vi "微波探针下压同步采集系统.vi"() -> ()   [LabVIEW 2024]
uses:
  <vilib>/Analysis/Matrix/Datatypes/RealMatrix.ctl
  <vilib>/Instr/_visa.llb/VISA Configure Serial Port (Instr).vi
  <vilib>/Utility/file.llb/Write Delimited Spreadsheet (DBL).vi
  BP_GAS/GAS.lvlib
  BP_GAS/VIs/GA Open.vi
  BP_GAS/VIs/GA Reset.vi
  BP_GAS/VIs/GA Axis On.vi
  BP_GAS/VIs/GA Prf Trap.vi
  BP_GAS/VIs/GA Set Trap Prm Single.vi
  BP_GAS/VIs/GA Set Vel.vi
  BP_GAS/VIs/GA Set Pos.vi
  BP_GAS/VIs/GA Get Prf Pos.vi
  BP_GAS/VIs/GA Stop.vi
  BP_GAS/VIs/GA Update.vi
  <vilib>/Analysis/Matrix/NI_Matrix.lvlib
panel:
  out "循环次数":T1
  in  "循环次数":dbl
  out "步骤":T1
  in  "启用":bool
  in  "Real Matrix":T2 caption="顺序移动"
  out "U":dbl
  out "Z":dbl
  out "Y":dbl
  out "X":dbl
  out "错误输出 2":errorcluster caption="错误输出"
  out "错误输出":errorcluster
  out "电容":dbl(graph)
  out "电容表":dbl(knob) scale=0.0..20.0
  out "电容(F)":dbl
  out "损耗因子表":dbl(knob) scale=0.0..10.0
  out "损耗因子":dbl(graph)
  out "损耗因子(F)":dbl
  in  "测试参数":u16(ring) items=["Ls-Rs", "Cp-D"]
  in  "复位":bool
  out "运动状态":bool
  out "error out 2":errorcluster caption="error out"
  in  "停止运动":bool
  in  "开始运动":bool
  out "毫秒计时":u32
  out "时间":u32(graph)
  out "采集状态":bool
  out "位移 2":T3 scale=-10000.0..10000.0
  out "位置":dbl(graph)
  out "位置(pluse)":dbl
  out "info":string="打开成功！\r\n复位成功！\r\n轴使能成功！\r\n模式设置成功！\r\n参数设置成功！\r\n速度设置成功！\r\n目标位置成功！\r\n启动成功！\r\n启动成功！\r\n启动成功！\r\n启动成功！\r\n启动成功！\r\n启动成功！\r\n启动成功！\r\n启动成功！\r\n"
  out "实际位置":dbl
  in  "目标位置(mm or °)":dbl
  in  "设定速度(μm/s)":dbl=1.0 format="%#_13g"
  in  "轴号":i16=3
  out "电感":dbl(graph)
  out "电阻表 3":dbl(knob) scale=0.0..20.0
  out "电感(H)":dbl
  out "电阻表 2":dbl(knob) scale=0.0..10.0
  out "电阻":dbl(graph)
  out "电阻(Ω)":dbl
  in  "Baud Rate":u32=9600
  in  "LCR数字电桥":refnum<visa-resource-name>="COM7"
  in  "保存数据":bool
  in  "压力归零":bool
  in  "清除图表":bool
  in  "开始采集":bool
  out "压力表":dbl(knob) scale=0.0..20.0
  out "压力":dbl(graph)
  out "压力(g)":dbl
  in  "stop bits (10: 1 bit) 2":u16(ring)=10 caption="停止位（10: 1位）" items=["1.0"=10, "1.5"=15, "2.0"=20]
  in  "timeout (10sec) 2":u32=10000 caption="超时（10秒）"
  in  "parity (0:none) 2":enum16{"None", "Odd", "Even", "Mark", "Space"}(ring) caption="奇偶（0:无）"
  in  "baud rate (9600) 2":u32=9600 caption="波特率(9600)"
  in  "data bits (8) 2":u16=8 caption="数据比特(8)" min=5 max=8 step=1
  in  "VISA resource name 2":refnum<visa-resource-name>="COM5" caption="压力串口"
  in  "读取间隔（毫秒）":u32=100
  in  "停止":bool
  # "XYZU：0.078125μm/pluse"
  # "位置       速度     延时(ms)"
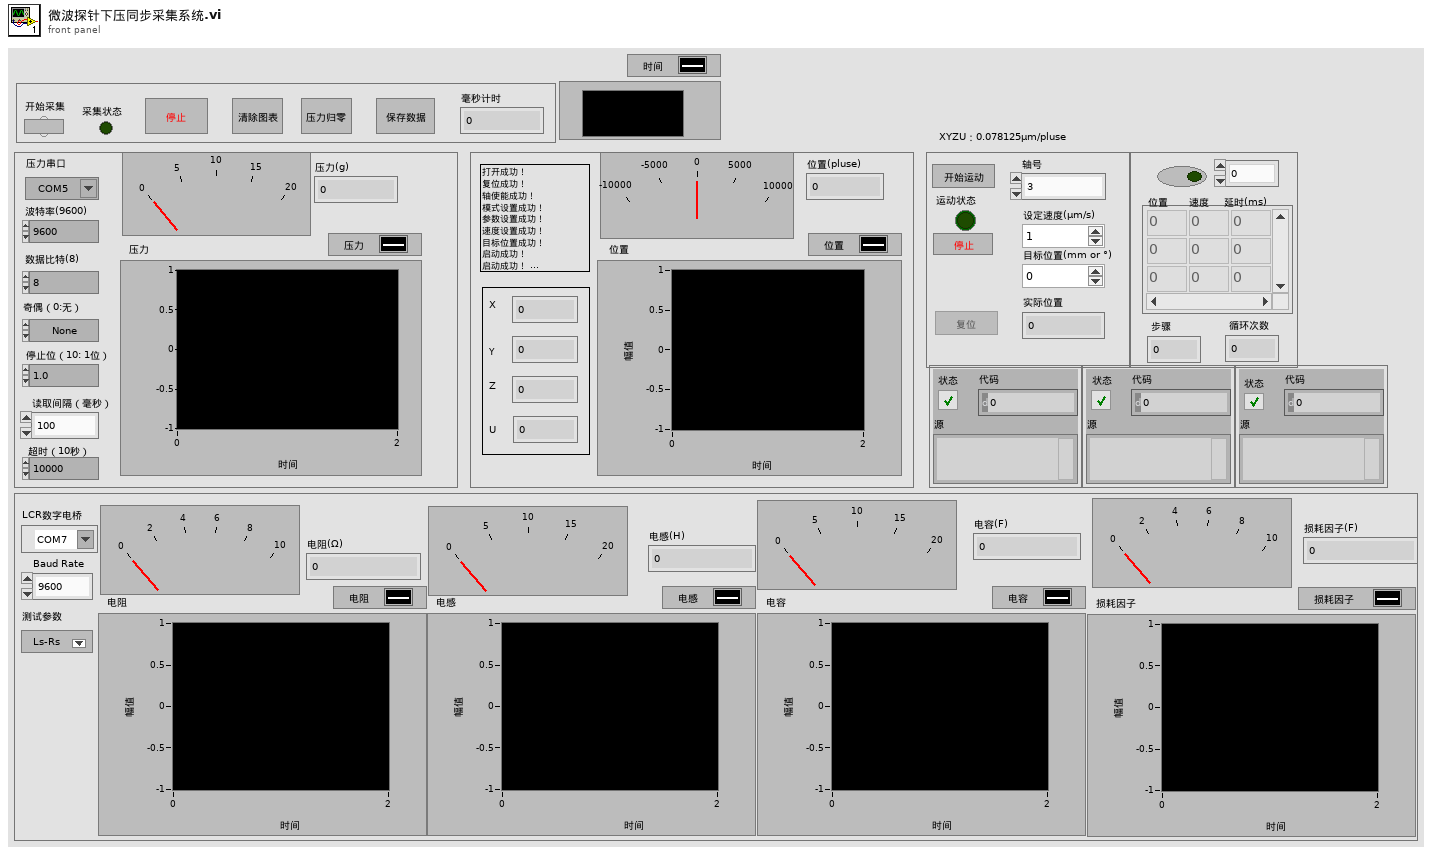
[diagram p1: front panel]
types:
  T1 = typedef "控件 3.ctl" = dbl
  T2 = typedef "NI_Matrix.lvlib/RealMatrix.ctl" = dbl[][]
  T3 = typedef "控件 1.ctl" = dbl
  T4 = enum8{"Enabled", "Disabled", "Disabled and Grayed Out"}
  T5 = cluster{"acc":dbl, "dec":dbl, "velStart":dbl, "smoothTime":i16}
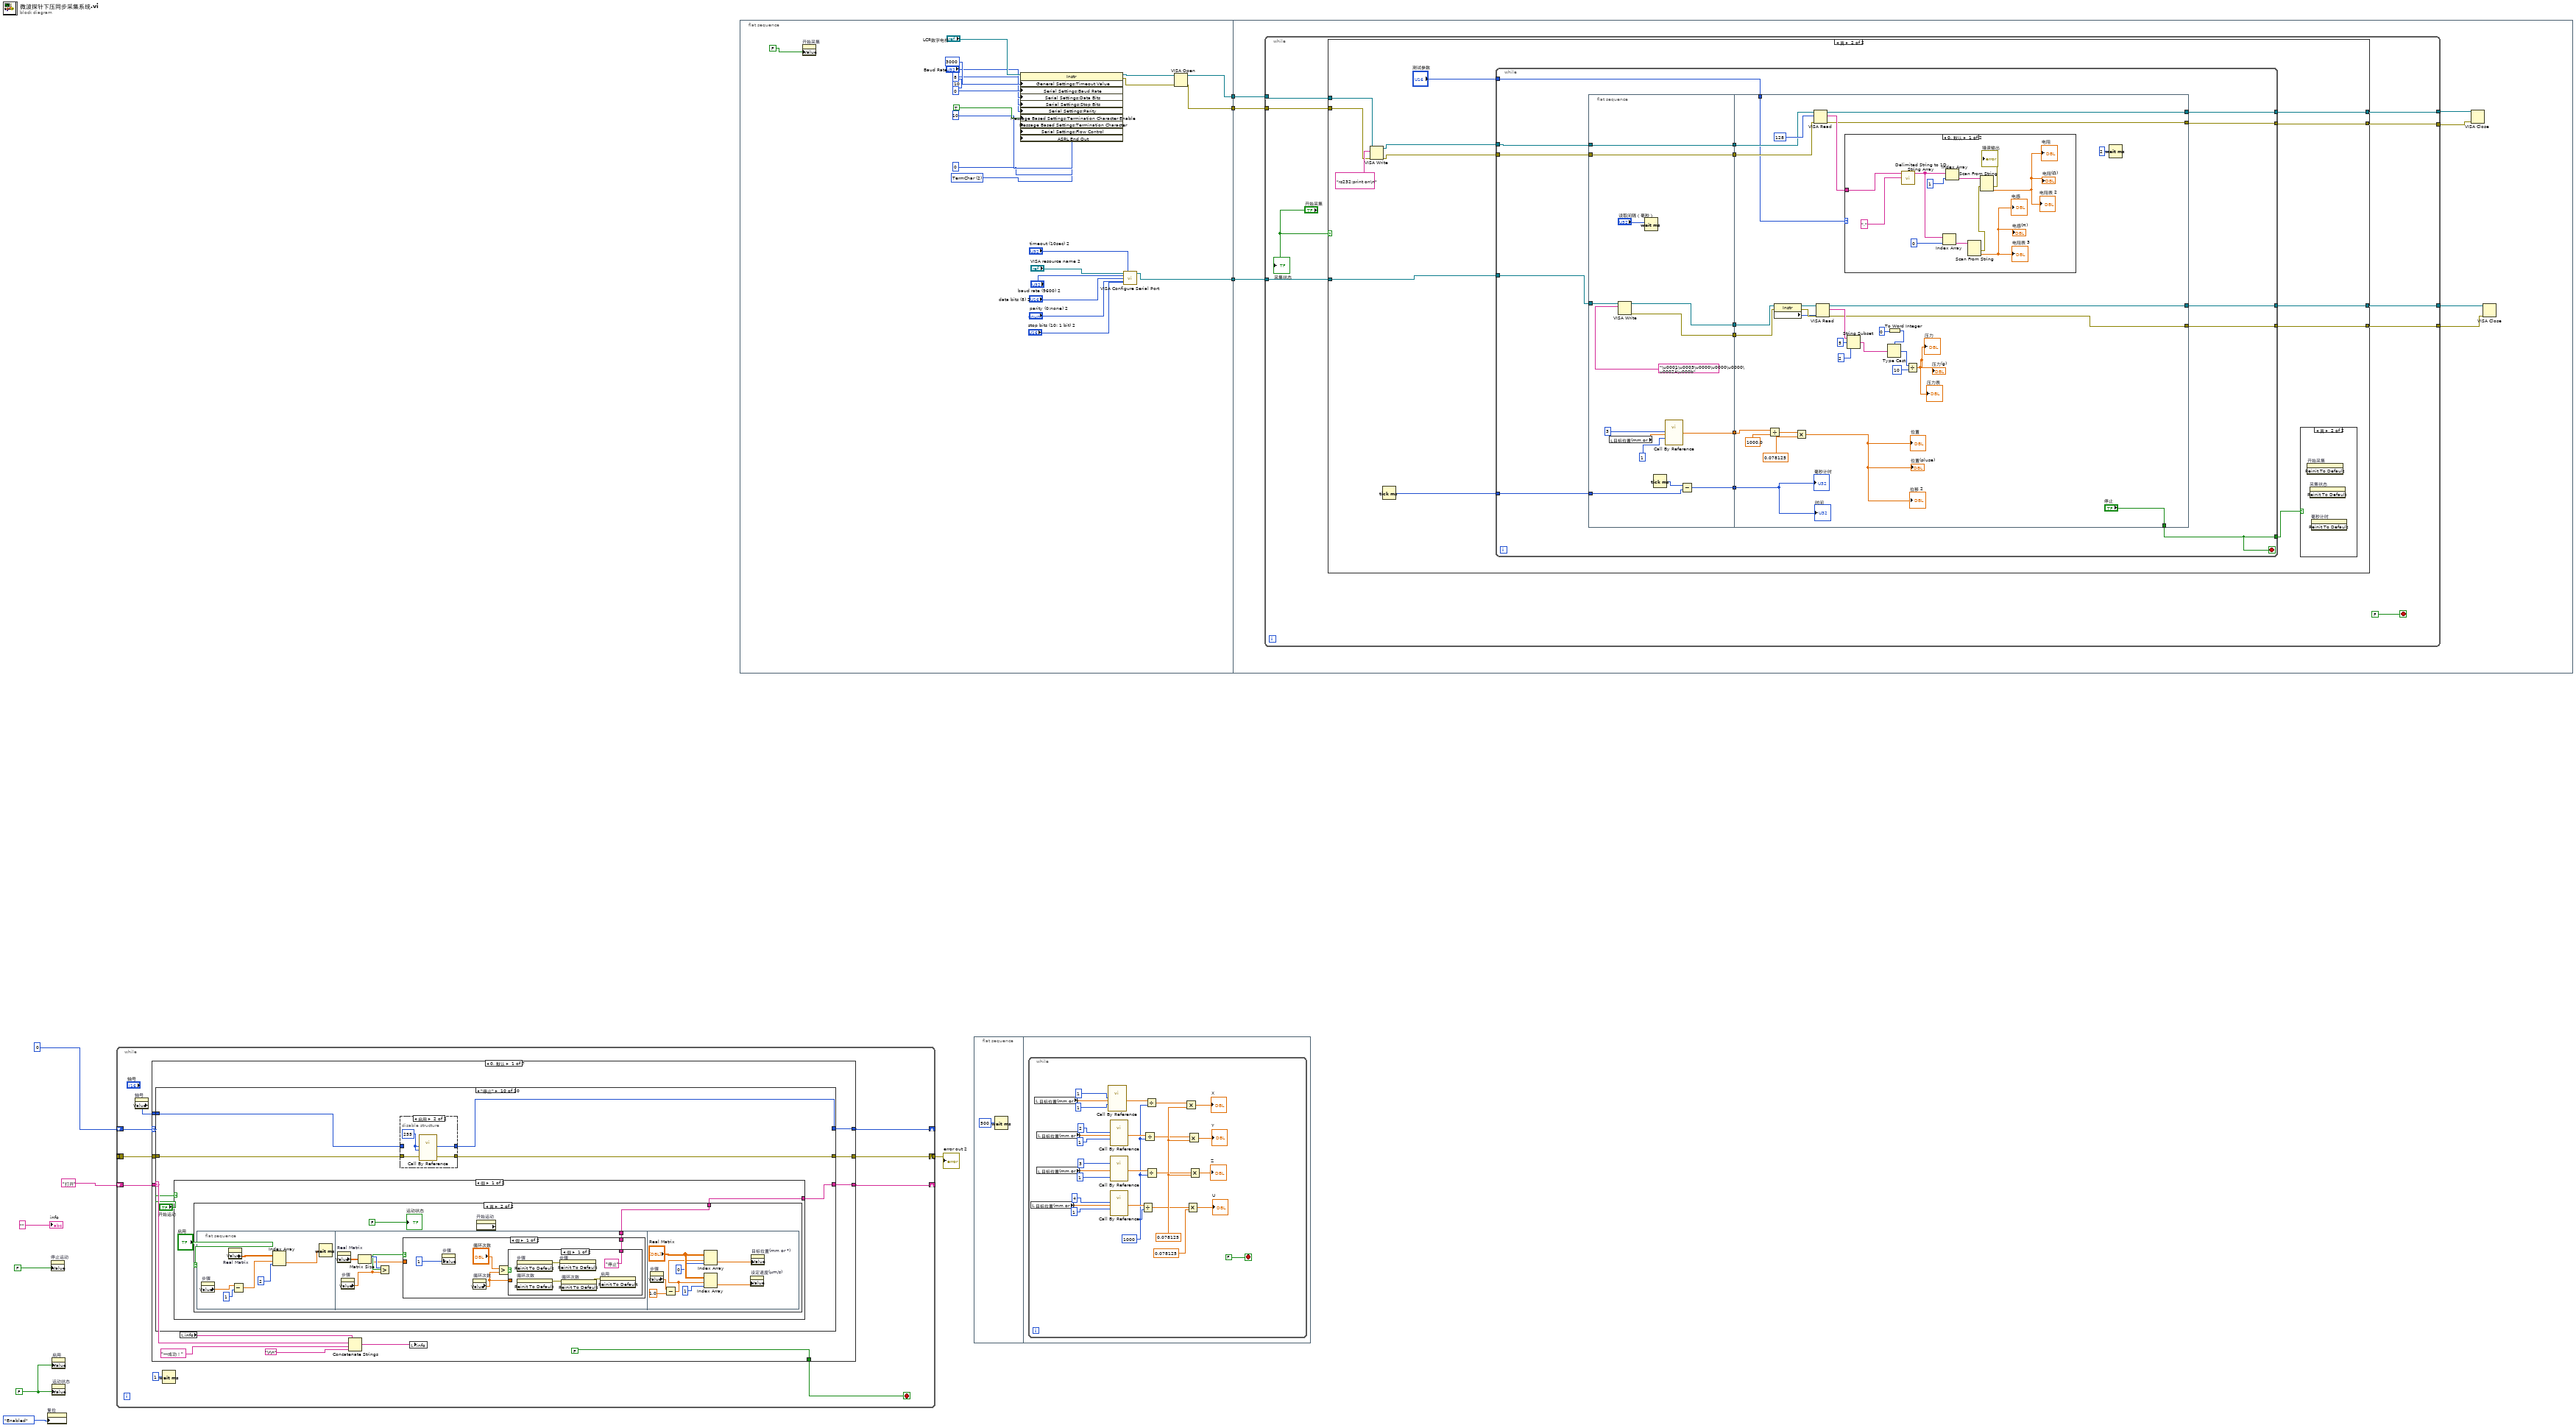
[diagram p0: block diagram]
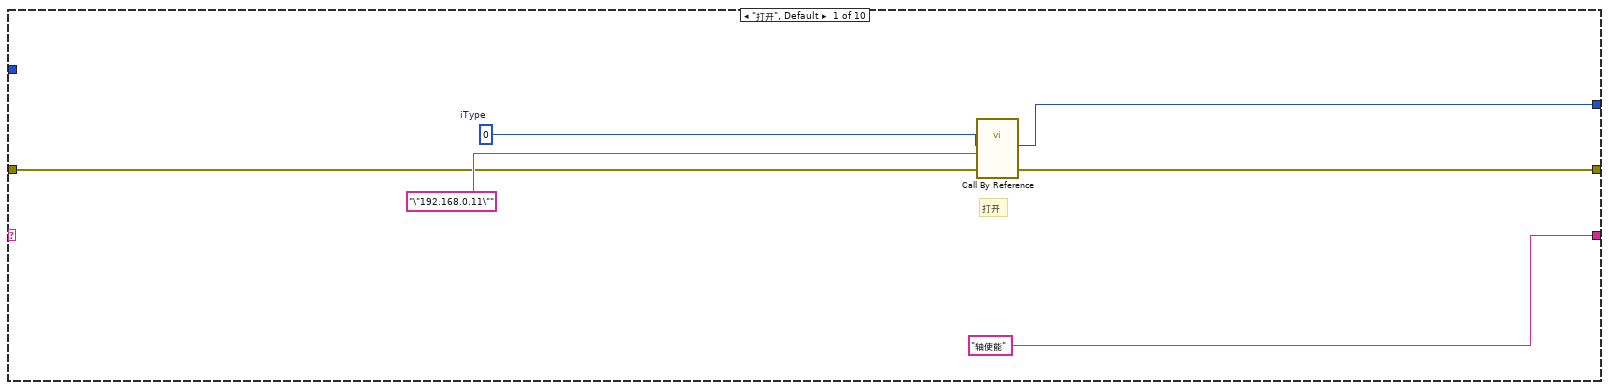
[diagram p2: hidden frame]
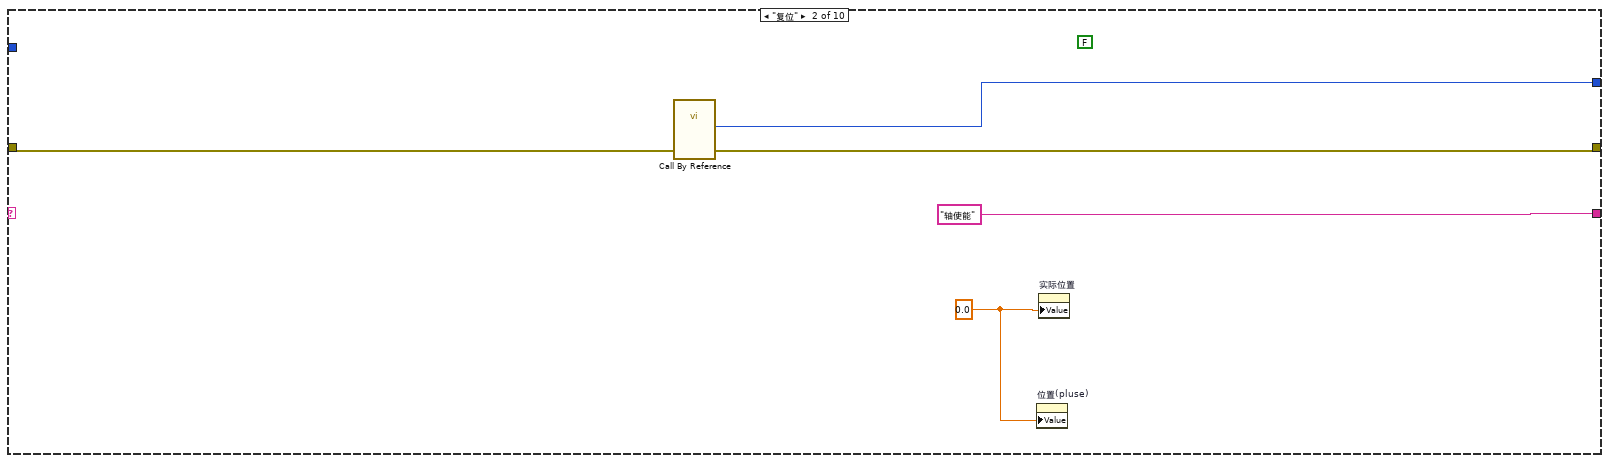
[diagram p3: hidden frame]
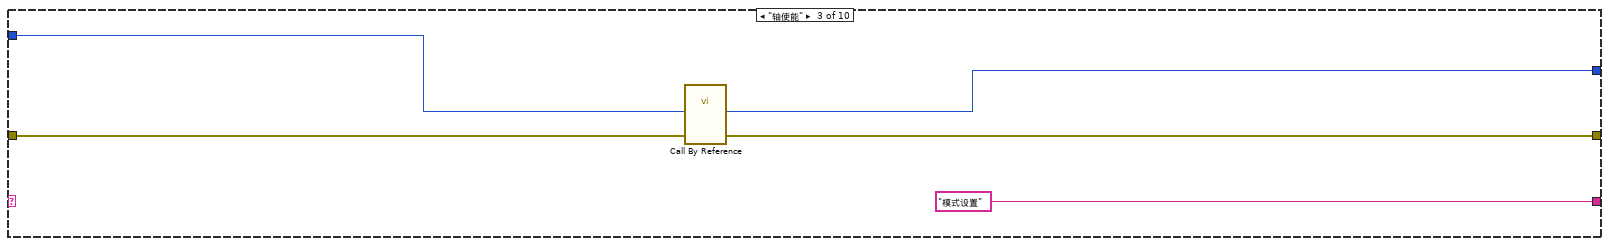
[diagram p4: hidden frame]
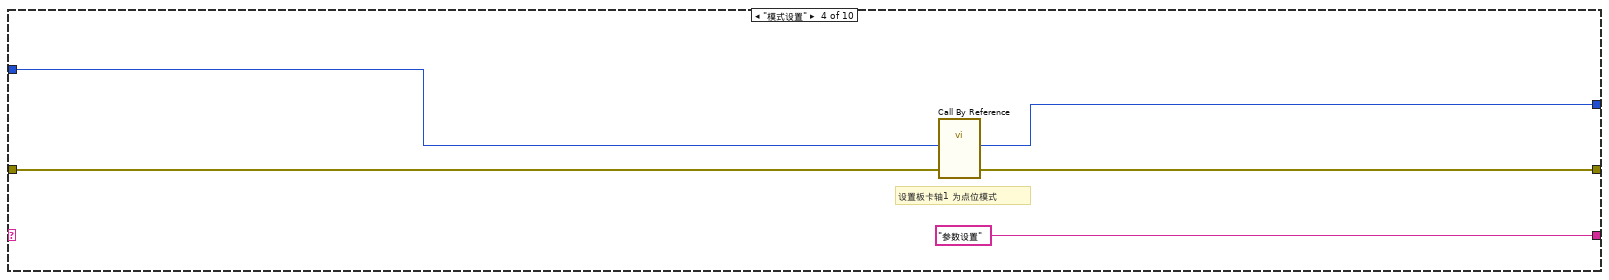
[diagram p5: hidden frame]
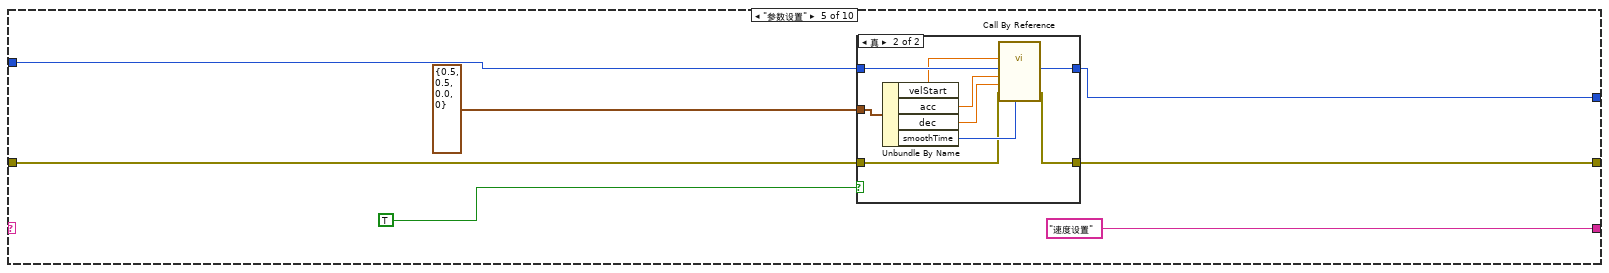
[diagram p6: hidden frame]
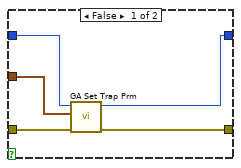
[diagram p7: hidden frame]
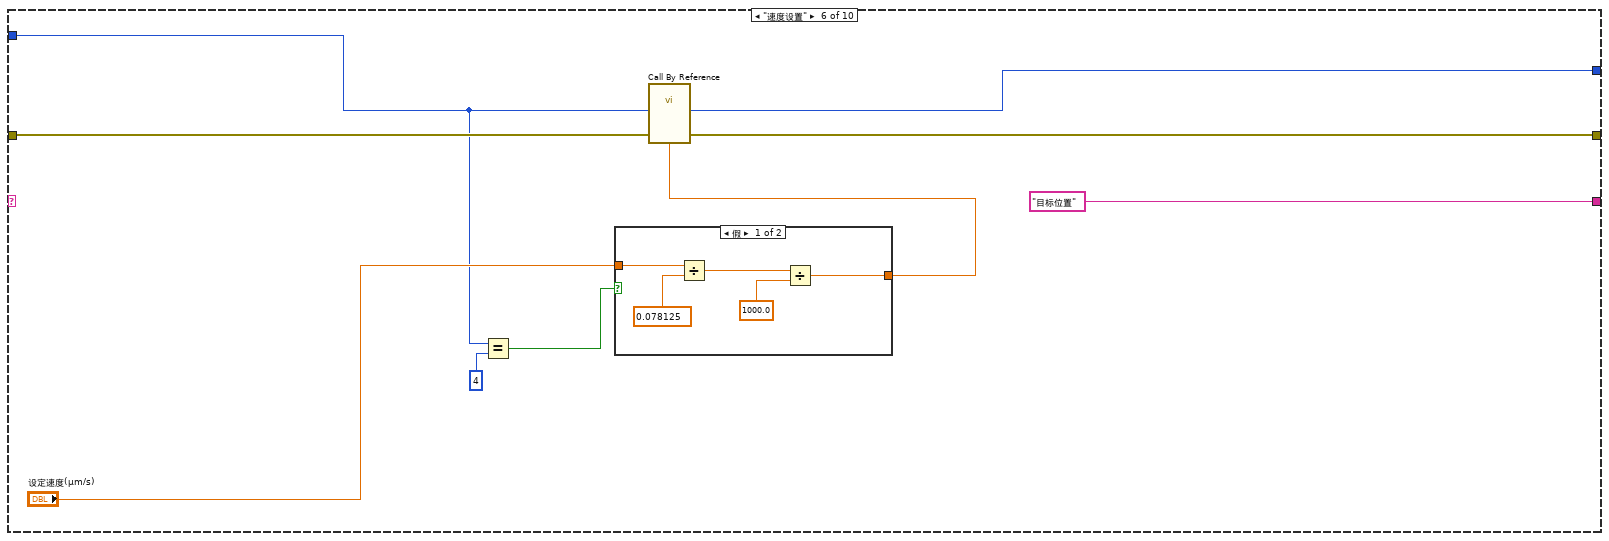
[diagram p8: hidden frame]
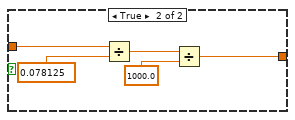
[diagram p9: hidden frame]
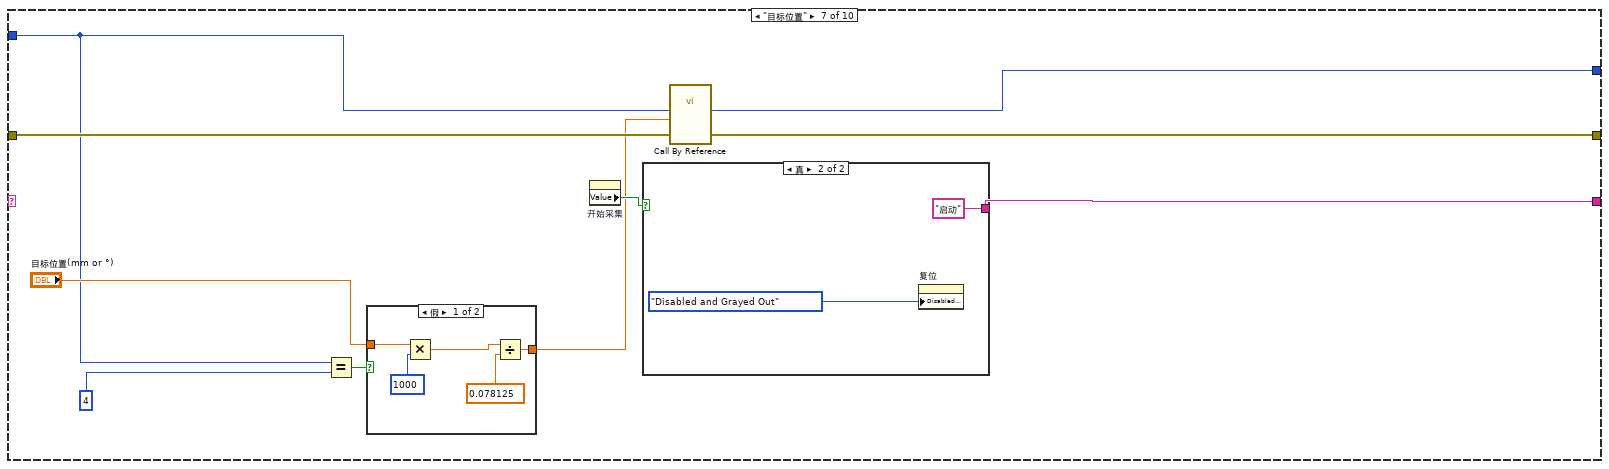
[diagram p10: hidden frame]
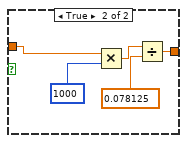
[diagram p11: hidden frame]
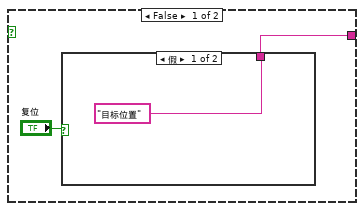
[diagram p12: hidden frame]
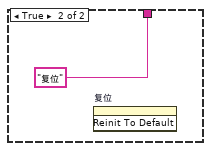
[diagram p13: hidden frame]
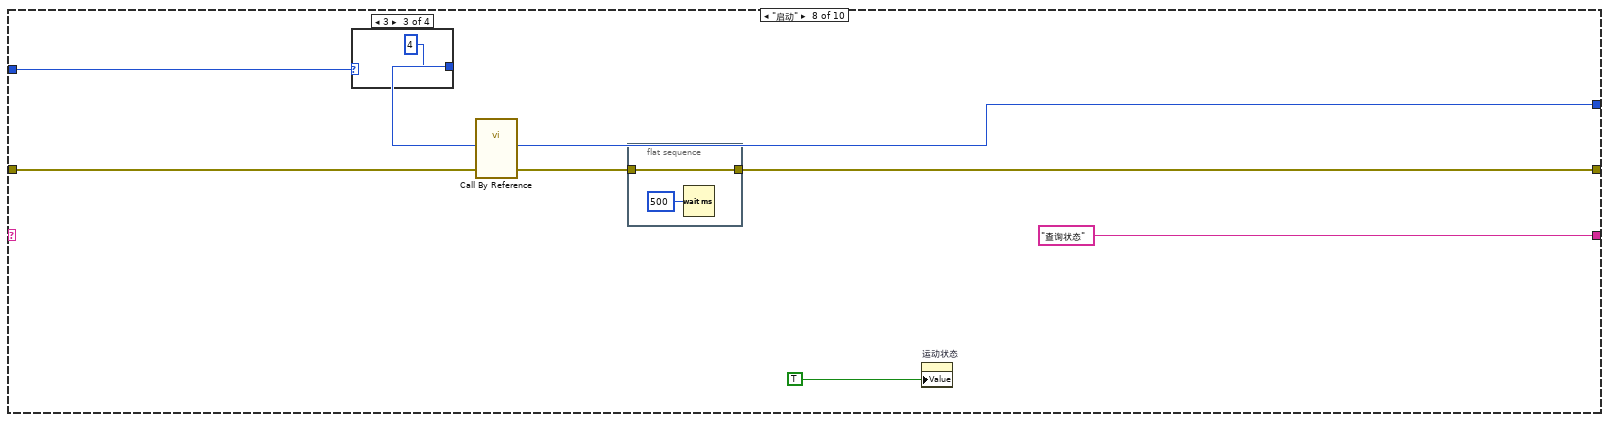
[diagram p14: hidden frame]
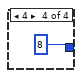
[diagram p17: hidden frame]
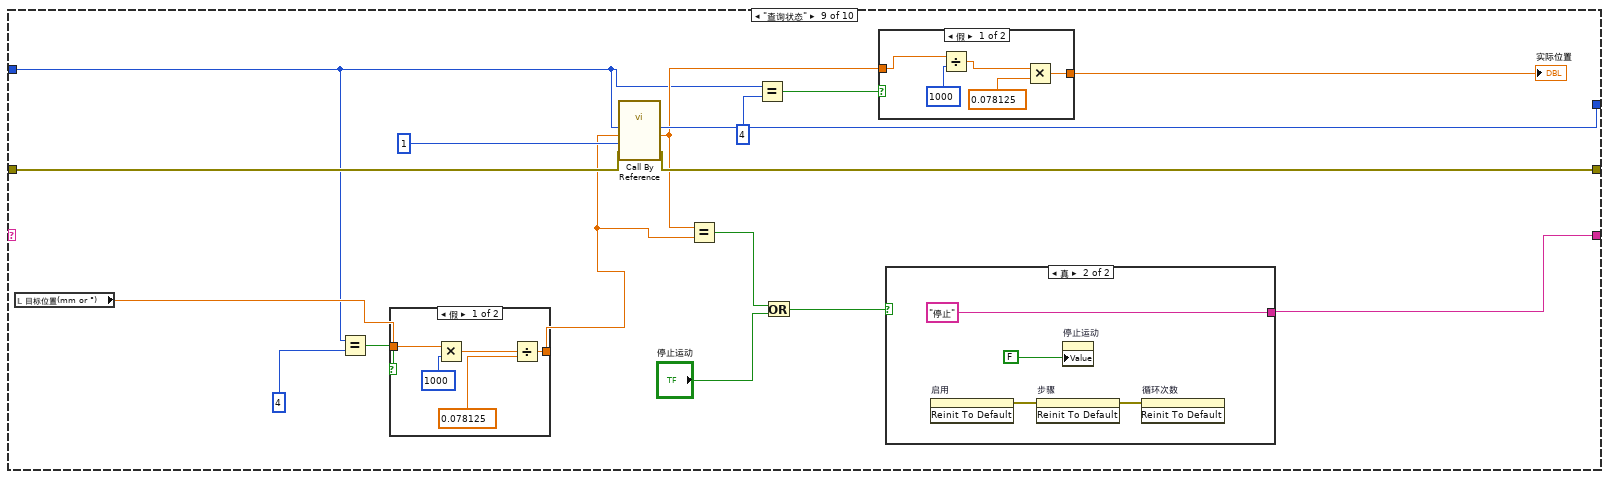
[diagram p18: hidden frame]
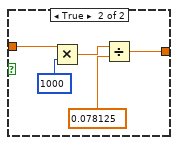
[diagram p19: hidden frame]
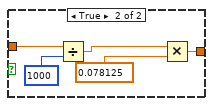
[diagram p20: hidden frame]
diagram:
  w1 = FALSE
  n1 = property on="复位" class="Bool"("DisabledEnum"=T4."Enabled" ("禁用")) -> ()  [unwired: 2 in, 2 out]
  n2 = property on="停止运动" class="Bool (严格)"("Value"=FALSE) -> ()  [unwired: 2 in, 2 out]
  n3 = property on="启用" class="Bool (严格)"("Value"=w1) -> ()  [unwired: 2 in, 2 out]
  n4 = property on="运动状态" class="Bool (严格)"("Value"=w1) -> ()  [unwired: 2 in, 2 out]
  n5 = while {
    shift-right: [w18] -> _
    shift-left: 0 -> [w19]
    shift-right: [w12] -> _
    shift-left: _ -> [w13]
    shift-right: [w16] -> _
    shift-left: "打开" -> [w15]
    tunnel: [w13] -> _
    tunnel: [w12] -> w3
    stop <- w11 stop-if-true
    n6 = property on="轴号" class="DigNum (严格)"() -> ("Value"=w14:i16)  [unwired: 2 in, 2 out]
    n7 = case shown="0, 默认" w19 {
      tunnel: [w30 0 0 0 0 0 0] -> w18
      tunnel: w13 -> [w29 w236 w243 w250 w257 w264 w271]
      tunnel: [w28 w236 w243 w250 w257 w264 w271] -> w12
      tunnel: w15 -> [w22 _ _ _ _ _ _]
      tunnel: [w23 "打开" "打开" "打开" "打开" "打开" "打开"] -> w16
      tunnel: w14 -> [w27 _ _ _ _ _ _]
      tunnel: [FALSE TRUE TRUE TRUE TRUE TRUE TRUE] -> w11
      frame 0, Default {
        n8 = case shown="\"停止\"" w22 {
          tunnel: [w32 w41 w44 w48 w52 w79 w99 w125 w147 w174] -> w30
          tunnel: w29 -> [w33 w39 w46 w50 w55 w81 w101 w124 w146 w179]
          tunnel: [w35 w40 w45 w49 w54 w80 w100 w121 w148 w178] -> w28
          tunnel: ["轴使能" "轴使能" "模式设置" "参数设置" "速度设置" "目标位置" w98 "查询状态" w144 w175] -> w23
          tunnel: w27 -> [_ _ w43 w47 w53 w76 w93 w120 w133 w177]
          frame "打开", Default {
            w36 = i16 0  # iType
            # "打开"
            n9 = call-by-ref "?"("error in (no error)"=w33, "cName"="\"192.168.0.11\"", "iType"=w36) -> ("error out"=w35:errorcluster, "function return"=w32:i32)  [unwired: 8 in, 3 out]
          }
          frame "复位" {
            (unwired) FALSE
            w37 = 0.0 ("实际位置")
            n10 = call-by-ref "?"("error in (no error)"=w39) -> ("error out"=w40:errorcluster, "function return"=w41:i32)  [unwired: 11 in, 2 out]
            n11 = property on="位置(pluse)" class="DigNum (严格)"("Value"=w37) -> ()  [unwired: 2 in, 2 out]
            n12 = property on="实际位置" class="DigNum (严格)"("Value"=w37) -> ()  [unwired: 2 in, 2 out]
          }
          frame "轴使能" {
            n13 = call-by-ref "?"("error in (no error)"=w46, "nAxisNum"=w43) -> ("error out"=w45:errorcluster, "function return"=w44:i32)  [unwired: 10 in, 2 out]
          }
          frame "模式设置" {
            # "设置板卡轴1 为点位模式"
            n14 = call-by-ref "?"("error in (no error)"=w50, "nAxisNum"=w47) -> ("error out"=w49:errorcluster, "function return"=w48:i32)  [unwired: 10 in, 2 out]
          }
          frame "参数设置" {
            n15 = case shown="真" TRUE ("单轴？") {
              tunnel: w55 -> [w63 w66]
              tunnel: w53 -> [w62 w71]
              tunnel: T5 {"acc"=0.5, "dec"=0.5, "velStart"=0.0, "smoothTime"=0} ("运动控制卡") -> [w61 w72]
              tunnel: [w60 w65] -> w54
              tunnel: [w59 w64] -> w52
              frame False {
                n16 = call "GA Set Trap Prm.vi"("error in (no error)"=w63, "pPrm"=w61, "nAxisNum"=w62) -> ("error out"=w60:errorcluster, "function return"=w59:i32)  [unwired: 6 in, 1 out]
              }
              frame True {
                n17 = Unbundle By Name(w72) -> ("velStart"=w67:dbl, "acc"=w69:dbl, "dec"=w68:dbl, "smoothTime"=w70:i16)
                n18 = call-by-ref "?"("dSmoothTime"=w70, "dVelStart"=w67, "error in (no error)"=w66, "dDec"=w68, "dAcc"=w69, "nAxisNum"=w71) -> ("error out"=w65:errorcluster, "function return"=w64:i32)  [unwired: 6 in, 2 out]
              }
            }
          }
          frame "速度设置" {
            n19 = Equal?(x=w76, y=i16 4) -> (x = y?=w74:bool)
            n20 = case shown="假" w74 {
              tunnel: [w82 w87] -> w73
              tunnel: "设定速度(μm/s)" -> [w85 w90]
              frame False {
                n21 = Divide(x=w85, y=0.078125) -> (x/y=w83:dbl)
                n22 = Divide(x=w83, y=1000.0) -> (x/y=w82:dbl)
              }
              frame True {
                n23 = Divide(x=w90, y=0.078125) -> (x/y=w89:dbl)
                n24 = Divide(x=w89, y=1000.0) -> (x/y=w87:dbl)
              }
            }
            n25 = call-by-ref "?"("error in (no error)"=w81, "vel"=w73, "nAxisNum"=w76) -> ("error out"=w80:errorcluster, "function return"=w79:i32)  [unwired: 9 in, 2 out]
          }
          frame "目标位置" {
            n26 = Equal?(x=w93, y=i16 4) -> (x = y?=w95:bool)
            n27 = case shown="假" w95 {
              tunnel: [w105 w110] -> w92
              tunnel: "目标位置(mm or °)" -> [w102 w108]
              frame False {
                n28 = Multiply(x=w102, y=1000) -> (x*y=w103:dbl)
                n29 = Divide(x=w103, y=0.078125) -> (x/y=w105:dbl)
              }
              frame True {
                n30 = Multiply(x=w108, y=1000) -> (x*y=w107:dbl)
                n31 = Divide(x=w107, y=0.078125) -> (x/y=w110:dbl)
              }
            }
            n32 = property on="开始采集" class="Bool (严格)"() -> ("Value"=w97:bool)  [unwired: 2 in, 2 out]
            n33 = case shown="真" w97 {
              tunnel: [w112 "启动"] -> w98
              frame False {
                n34 = case shown="假" "复位" {
                  tunnel: ["目标位置" "复位"] -> w112
                  frame False {
                  }
                  frame True {
                    n35 = invoke on="复位" class="Bool" method="Reinit To Default"() -> ()  [unwired: 3 in, 3 out]
                  }
                }
              }
              frame True {
                n36 = property on="复位" class="Bool"("DisabledEnum"=T4."Disabled and Grayed Out" ("禁用")) -> ()  [unwired: 2 in, 2 out]
              }
            }
            n37 = call-by-ref "?"("error in (no error)"=w101, "pos"=w92, "nAxisNum"=w93) -> ("error out"=w100:errorcluster, "function return"=w99:i32)  [unwired: 9 in, 2 out]
          }
          frame "启动" {
            n38 = case shown="3" w120 {
              selector: w120 -> [w126 w127 _ _]
              tunnel: [w126 w127 4 8] -> w119
              frame 1, Default {
              }
              frame 2 {
              }
              frame 3 {
              }
              frame 4 {
              }
            }
            n39 = call-by-ref "?"("error in (no error)"=w124, "mask"=w119) -> ("error out"=w122:errorcluster, "function return"=w125:i32)  [unwired: 10 in, 2 out]
            n40 = flat-sequence {
              tunnel: w122 -> [w131]
              tunnel: [w131] -> w121
              frame #0 {
                n41 = Wait (ms)(milliseconds to wait=u32 500 ("等待时间（毫秒）")) -> ()  [unwired: 1 out]
              }
            }
            n42 = property on="运动状态" class="Bool (严格)"("Value"=TRUE) -> ()  [unwired: 2 in, 2 out]
          }
          frame "查询状态" {
            n43 = local read "目标位置(mm or °)"() -> (w134:dbl)
            n44 = Equal?(x=w133, y=i16 4) -> (x = y?=w135:bool)
            n45 = case shown="假" w135 {
              tunnel: [w152 w157] -> w132
              tunnel: w134 -> [w150 w154]
              frame False {
                n46 = Multiply(x=w150, y=1000) -> (x*y=w149:dbl)
                n47 = Divide(x=w149, y=0.078125) -> (x/y=w152:dbl)
              }
              frame True {
                n48 = Multiply(x=w154, y=1000) -> (x*y=w155:dbl)
                n49 = Divide(x=w155, y=0.078125) -> (x/y=w157:dbl)
              }
            }
            n50 = call-by-ref "?"("error in (no error)"=w146, "nCount"=i16 1, "pValue"=w132, "nAxisNum"=w133) -> ("error out"=w148:errorcluster, "pValue out"=w139:dbl, "function return"=w147:i32)  [unwired: 6 in, 3 out]
            n51 = Equal?(x=w139, y=w132) -> (x = y?=w143:bool)
            n52 = Equal?(x=w133, y=i16 4) -> (x = y?=w140:bool)
            n53 = Or(x=w143, y="停止运动") -> (x .or. y?=w141:bool)
            n54 = case shown="假" w140 {
              tunnel: [w162 w167] -> w137
              tunnel: w139 -> [w159 w164]
              frame False {
                n55 = Divide(x=w159, y=1000) -> (x/y=w160:dbl)
                n56 = Multiply(x=w160, y=0.078125) -> (x*y=w162:dbl)
              }
              frame True {
                n57 = Divide(x=w164, y=1000) -> (x/y=w165:dbl)
                n58 = Multiply(x=w165, y=0.078125) -> (x*y=w167:dbl)
              }
            }
            "实际位置" <- w137
            n59 = case shown="真" w141 {
              tunnel: ["查询状态" "停止"] -> w144
              frame False {
              }
              frame True {
                n60 = invoke on="启用" class="Bool (严格)" method="Reinit To Default"() -> (error out=w171:errorcluster)  [unwired: 3 in, 2 out]
                n61 = invoke on="步骤" class="DigNum (严格)" method="Reinit To Default"(error in=w171) -> (error out=w170:errorcluster)  [unwired: 2 in, 2 out]
                n62 = property on="停止运动" class="Bool (严格)"("Value"=FALSE ("停止运动")) -> ()  [unwired: 2 in, 2 out]
                n63 = invoke on="循环次数" class="DigNum (严格)" method="Reinit To Default"(error in=w170) -> ()  [unwired: 2 in, 3 out]
              }
            }
          }
          frame "停止" {
            n64 = case shown="假" "开始运动" {
              tunnel: [w181 "轴使能"] -> w175
              frame False {
                n65 = case shown="真" "启用" {
                  tunnel: ["停止" w184] -> w181
                  frame False {
                    n66 = property on="开始运动" class="Bool"("DisabledEnum"=T4."Enabled" ("禁用")) -> ()  [unwired: 2 in, 2 out]
                  }
                  frame True {
                    n67 = flat-sequence {
                      tunnel: [w192] -> w184
                      frame #0 {
                        n68 = property on="步骤" class="DigNum (严格)"() -> ("Value"=w188:T1)  [unwired: 2 in, 2 out]
                        n69 = property on="Real Matrix" class="Arr (严格)"() -> ("Value"=w191:T2)  [unwired: 2 in, 2 out]
                        n70 = Subtract(x=w188, y=1) -> (x-y=w186:T1)
                        n71 = Index Array(array=w191, index (row)=w186, index (col)=u32 2 ("等待时间（毫秒）")) -> (element=w189:dbl)
                        n72 = Wait (ms)(milliseconds to wait=w189) -> ()  [unwired: 1 out]
                      }
                      frame #1 {
                        n73 = property on="Real Matrix" class="Arr (严格)"() -> ("Value"=w196:T2)  [unwired: 2 in, 2 out]
                        n74 = property on="步骤" class="DigNum (严格)"() -> ("Value"=w193:T1)  [unwired: 2 in, 2 out]
                        n75 = Matrix Size(0:w196) -> (1:w195:i32)  [unwired: 1 out]
                        n76 = Greater?(x=w195, y=w193) -> (0:w194:bool)
                        n77 = case shown="假" w194 {
                          tunnel: w193 -> [_ w213]
                          tunnel: [w197 "轴使能"] -> w192
                          frame False {
                            n78 = property on="步骤" class="DigNum (严格)"("Value"=1) -> ()  [unwired: 2 in, 2 out]
                            n79 = property on="循环次数" class="DigNum (严格)"() -> ("Value"=w198:T1)  [unwired: 2 in, 2 out]
                            n80 = Greater?(x="循环次数", y=w198) -> (0:w200:bool)
                            n81 = case shown="假" w200 {
                              tunnel: w198 -> [_ w209]
                              tunnel: ["停止" "轴使能"] -> w197
                              frame False {
                                n82 = invoke on="步骤" class="DigNum (严格)" method="Reinit To Default"() -> (error out=w203:errorcluster)  [unwired: 3 in, 2 out]
                                n83 = invoke on="循环次数" class="DigNum (严格)" method="Reinit To Default"() -> (error out=w202:errorcluster)  [unwired: 3 in, 2 out]
                                n84 = invoke on="步骤" class="DigNum (严格)" method="Reinit To Default"(error in=w203) -> ()  [unwired: 2 in, 3 out]
                                n85 = invoke on="循环次数" class="DigNum (严格)" method="Reinit To Default"(error in=w202) -> (error out=w204:errorcluster)  [unwired: 2 in, 2 out]
                                n86 = invoke on="启用" class="Bool (严格)" method="Reinit To Default"(error in=w204) -> ()  [unwired: 2 in, 3 out]
                              }
                              frame True {
                                n87 = Add(x=1, y=w209) -> (x+y=→"循环次数":T1)
                              }
                            }
                          }
                          frame True {
                            n88 = Add(x=w213, y=1) -> (x+y=→"步骤":T1)
                          }
                        }
                      }
                      frame #2 {
                        n89 = property on="步骤" class="DigNum (严格)"() -> ("Value"=w216:T1)  [unwired: 2 in, 2 out]
                        n90 = Subtract(x=w216, y=T1 1.0) -> (x-y=w214:T1)
                        n91 = Index Array(array="Real Matrix", index (row)=w214, index (col)=1) -> (element=w219:dbl)
                        n92 = Index Array(array="Real Matrix", index (row)=w214, index (col)=0) -> (element=w220:dbl)
                        n93 = property on="设定速度(μm/s)" class="DigNum (严格)"("Value"=w219) -> ()  [unwired: 2 in, 2 out]
                        n94 = property on="目标位置(mm or °)" class="DigNum (严格)"("Value"=w220) -> ()  [unwired: 2 in, 2 out]
                      }
                    }
                    n95 = property on="开始运动" class="Bool" props=["DisabledEnum"]() -> ()  [unwired: 2 in, 3 out]
                    "运动状态" <- FALSE
                  }
                }
              }
              frame True {
                n96 = invoke on="开始运动" class="Bool" method="Reinit To Default"() -> ()  [unwired: 3 in, 3 out]
              }
            }
            n97 = disable-structure shown="启用" {
              disable-tunnel: w179 -> [w226 w230]
              disable-tunnel: [w225 w228] -> w178
              disable-tunnel: w177 -> [w224 _]
              disable-tunnel: [w223 w229] -> w174
              frame Disabled {
                n98 = call "GA Axis Off.vi"("error in (no error)"=w226, "nAxisNum"=w224) -> ("error out"=w225:errorcluster, "function return"=w223:i32)  [unwired: 8 in]
              }
              frame Enabled {
                w227 = 255 ("lMask")
                n99 = call-by-ref "?"("error in (no error)"=w230, "lOption"=w227, "lMask"=w227) -> ("error out"=w228:errorcluster, "function return"=w229:i32)  [unwired: 9 in, 2 out]
              }
            }
          }
        }
        n100 = local read "info"() -> (w26:string)
        n101 = Concatenate Strings(w26, w22, "---成功！" ("字符串"), "\r\n") -> (w24:string)
        n102 = local write "info"(w24) -> ()
      }
      frame 1 {
        w232 = "执行失败!" ("消息")
        n103 = local read "info"() -> (w233:string)
        n104 = Concatenate Strings(w233, w232) -> (w234:string)
        n105 = One Button Dialog(message=w232) -> ()  [unwired: 1 in, 1 out]
        n106 = local write "info"(w234) -> ()
      }
      frame 2 {
        w239 = "版本不支持该API" ("消息")
        n107 = local read "info"() -> (w240:string)
        n108 = One Button Dialog(message=w239) -> ()  [unwired: 1 in, 1 out]
        n109 = Concatenate Strings(w240, w239) -> (w241:string)
        n110 = local write "info"(w241) -> ()
      }
      frame 7 {
        w246 = "参数错误！检查参数配置是否合理！" ("消息")
        n111 = local read "info"() -> (w247:string)
        n112 = One Button Dialog(message=w246) -> ()  [unwired: 1 in, 1 out]
        n113 = Concatenate Strings(w247, w246) -> (w248:string)
        n114 = local write "info"(w248) -> ()
      }
      frame -6 {
        w253 = "打开控制器失败!\n检查串口或者网口IP配置是否正确。" ("消息")
        n115 = local read "info"() -> (w254:string)
        n116 = One Button Dialog(message=w253) -> ()  [unwired: 1 in, 1 out]
        n117 = Concatenate Strings(w254, w253) -> (w255:string)
        n118 = local write "info"(w255) -> ()
      }
      frame -1 {
        w260 = "通讯失败！确认接线是否牢靠!" ("消息")
        n119 = local read "info"() -> (w261:string)
        n120 = One Button Dialog(message=w260) -> ()  [unwired: 1 in, 1 out]
        n121 = Concatenate Strings(w261, w260) -> (w262:string)
        n122 = local write "info"(w262) -> ()
      }
      frame -7 {
        w267 = "运动控制器无响应！检查运动控制器是否正确连接、是否打开！" ("消息")
        n123 = local read "info"() -> (w268:string)
        n124 = Concatenate Strings(w268, w267) -> (w269:string)
        n125 = local write "info"(w269) -> ()
        n126 = One Button Dialog(message=w267) -> ()  [unwired: 1 in, 1 out]
      }
    }
    n127 = Wait (ms)(milliseconds to wait=u32 1 ("等待时间（毫秒）")) -> ()  [unwired: 1 out]
  }
  "error out 2" <- w3
  n128 = flat-sequence {
    tunnel: [w288] -> w10
    tunnel: [w276] -> w9
    tunnel: [w275] -> w8
    tunnel: w10 -> [w301]
    tunnel: w9 -> [w300]
    tunnel: w8 -> [w299]
    frame #0 {
      w283 = u16 2 items=["None", "Last Bit", "TermChar", "Break"] ("Serial Settings:End Mode for Writes")
      n129 = property on="开始采集" class="Bool (严格)"("Value"=FALSE) -> ()  [unwired: 2 in, 2 out]
      n130 = property class="Instr"(reference="LCR数字电桥", "General Settings:Timeout Value"=u32 3000, "Serial Settings:Baud Rate"="Baud Rate", "Serial Settings:Data Bits"=u16 8, "Serial Settings:Stop Bits"=u16 10, "Serial Settings:Parity"=u16 0, "Message Based Settings:Termination Character Enable"=TRUE ("TermChar En"), "Message Based Settings:Termination Character"=u8 10, "Serial Settings:Flow Control"=u16 0, "ASRL End Out"=w283) -> (reference out=w277:refnum<visa-resource-name>, error out=w274:errorcluster)  [unwired: 1 in]
      n131 = call-poly "VISA Configure Serial Port"("VISA resource name"="VISA resource name 2", "timeout (10sec)"="timeout (10sec) 2", "baud rate (9600)"="baud rate (9600) 2", "data bits (8)"="data bits (8) 2", "parity (0:none)"="parity (0:none) 2", "stop bits (10: 1 bit)"="stop bits (10: 1 bit) 2") -> ("VISA resource name out"=w288:refnum<visa-resource-name>)  [unwired: 8 in, 1 out]
      n132 = VISA Open(error in (no error)=w274, VISA resource name=w277) -> (VISA resource name=w276:refnum<visa-resource-name>, error out=w275:errorcluster)  [unwired: 3 in]
    }
    frame #1 {
      n133 = while {
        tunnel: w301 -> [w310]
        tunnel: w300 -> [w308]
        tunnel: w299 -> [w309]
        tunnel: [w307] -> w298
        tunnel: [w306] -> w297
        tunnel: [w305] -> w296
        tunnel: [w302] -> w295
        stop <- FALSE stop-if-true
        n134 = case shown="真" "开始采集" {
          tunnel: [w314 w355] -> w305
          tunnel: w310 -> [w315 w357]
          tunnel: w309 -> [_ w363]
          tunnel: w308 -> [w311 w362]
          tunnel: [w311 w356] -> w307
          tunnel: [_ w359] -> w306
          tunnel: [_ w353] -> w302
          frame False {
            (unwired) FALSE ("停止")
            n135 = case shown="假" "压力归零" {
              tunnel: w315 -> [w328 w331]
              tunnel: [w328 w329] -> w314
              frame False {
              }
              frame True {
                n136 = flat-sequence {
                  tunnel: w331 -> [w333]
                  tunnel: [w332] -> w330
                  tunnel: w330 -> [w339]
                  tunnel: [w336] -> w329
                  frame #0 {
                    n137 = VISA Write(VISA resource name=w333, write buffer="\u0001\u0010\u0000\u0000\u0000\u0002\u0004\u0000\u0000\u0000\u0000ó¯" ("写入缓冲区")) -> (VISA resource name out=w332:refnum<visa-resource-name>)  [unwired: 1 in, 2 out]
                  }
                  frame #1 {
                    n138 = VISA Write(VISA resource name=w339, write buffer="\u0001\u0003\u0000\u0000\u0000\u0002Ä\u000b" ("写入缓冲区")) -> (VISA resource name out=w338:refnum<visa-resource-name>, error out=w337:errorcluster)  [unwired: 1 in, 1 out]
                    n139 = property class="Instr"(reference=w338, error in=w337) -> (reference out=w351:refnum<visa-resource-name>, error out=w342:errorcluster, "Serial Settings:Number of Bytes at Serial Port"=w350:u32)
                    n140 = VISA Read(VISA resource name=w351, byte count=w350, error in (no error)=w342) -> (VISA resource name out=w336:refnum<visa-resource-name>, read buffer=w341:string)  [unwired: 2 out]
                    n141 = String Subset(string=w341, offset (0)=5 ("偏移量(0)"), length (rest)=2 ("长度（剩余）")) -> (substring=w347:string)
                    n142 = To Word Integer(number=0) -> (16bit integer=w345:i16)
                    n143 = Type Cast(type=w345, x=w347) -> (*(type *) &x=w344:i16)
                    n144 = Divide(x=w344, y=i16 10) -> (x/y=w335:dbl)
                    n145 = property on="压力(g)" class="DigNum (严格)"("Value"=w335) -> ()  [unwired: 2 in, 2 out]
                    n146 = property on="压力表" class="Knob (严格)"("Value"=w335) -> ()  [unwired: 2 in, 2 out]
                  }
                }
              }
            }
            n147 = case shown="假" "清除图表" {
              frame False {
              }
              frame True {
                w352 = dbl[] [] ("历史数据")
                n148 = property on="压力" class="WFChart (严格)"("History Data"=w352) -> ()  [unwired: 2 in, 2 out]
                n149 = property on="电感" class="WFChart (严格)"("History Data"=w352) -> ()  [unwired: 2 in, 2 out]
                n150 = property on="电阻" class="WFChart (严格)"("History Data"=w352) -> ()  [unwired: 2 in, 2 out]
                n151 = property on="位置" class="WFChart (严格)"("History Data"=w352) -> ()  [unwired: 2 in, 2 out]
                n152 = property on="时间" class="WFChart (严格)"("History Data"=w352) -> ()  [unwired: 2 in, 2 out]
                n153 = property on="电容" class="WFChart (严格)"("History Data"=w352) -> ()  [unwired: 2 in, 2 out]
                n154 = property on="损耗因子" class="WFChart (严格)"("History Data"=w352) -> ()  [unwired: 2 in, 2 out]
              }
            }
            n155 = case shown="假" "保存数据" {
              frame False {
              }
              frame True {
                n156 = property on="时间" class="WFChart (严格)"() -> ("History Data"=w318:u32[])  [unwired: 2 in, 2 out]
                n157 = property on="压力" class="WFChart (严格)"() -> ("History Data"=w324:dbl[])  [unwired: 2 in, 2 out]
                n158 = property on="位置" class="WFChart (严格)"() -> ("History Data"=w323:dbl[])  [unwired: 2 in, 2 out]
                n159 = property on="电阻" class="WFChart (严格)"() -> ("History Data"=w322:dbl[])  [unwired: 2 in, 2 out]
                n160 = property on="电感" class="WFChart (严格)"() -> ("History Data"=w321:dbl[])  [unwired: 2 in, 2 out]
                n161 = property on="电容" class="WFChart (严格)"() -> ("History Data"=w320:dbl[])  [unwired: 2 in, 2 out]
                n162 = property on="损耗因子" class="WFChart (严格)"() -> ("History Data"=w319:dbl[])  [unwired: 2 in, 2 out]
                n163 = Build Array(w318, w324, w323, w322, w321, w320, w319) -> (w326:dbl[][])
                n164 = Transpose Matrix(1:w326) -> (0:w325:dbl[][])
                n165 = call-poly <vilib>:"Write Delimited Spreadsheet.vi"("format (%.3f)"="%.20f", "2D data"=w325, "delimiter (\\t)"="," ("delimiter (\\t)")) -> ()  [unwired: 11 in, 2 out]
              }
            }
          }
          frame True {
            n166 = VISA Write(VISA resource name=w362, write buffer="rs232:print on\n" ("command"), error in (no error)=w363) -> (VISA resource name out=w360:refnum<visa-resource-name>, error out=w361:errorcluster)  [unwired: 1 out]
            n167 = Tick Count (ms)() -> (millisecond timer value=w365:u32)
            n168 = while {
              tunnel: [w371] -> w353
              tunnel: w365 -> [w381]
              tunnel: w361 -> [w378]
              tunnel: w360 -> [w376]
              tunnel: [w368] -> w359
              tunnel: "测试参数" -> [w367]
              tunnel: w357 -> [w380]
              tunnel: [w366] -> w354
              tunnel: [w370] -> w355
              tunnel: [w369] -> w356
              stop <- w366 stop-if-true
              n169 = flat-sequence {
                tunnel: w381 -> [w391]
                tunnel: w380 -> [w390]
                tunnel: w376 -> [w387]
                tunnel: [w387] -> w379
                tunnel: w378 -> [w386]
                tunnel: [w386] -> w377
                tunnel: [w385] -> w375
                tunnel: [w384] -> w374
                tunnel: [w383] -> w373
                tunnel: [w382] -> w372
                tunnel: ["停止"] -> w366
                tunnel: w379 -> [w411]
                tunnel: w377 -> [w410]
                tunnel: w375 -> [w409]
                tunnel: w374 -> [w408]
                tunnel: w373 -> [w398]
                tunnel: w372 -> [w407]
                tunnel: [w406] -> w371
                tunnel: [w405] -> w370
                tunnel: [w404] -> w369
                tunnel: [w403] -> w368
                tunnel: w367 -> [w402]
                frame #0 {
                  n170 = local read "目标位置(mm or °)"() -> (w394:dbl)
                  n171 = VISA Write(VISA resource name=w390, write buffer="\u0001\u0003\u0000\u0000\u0000\u0002Ä\u000b" ("写入缓冲区")) -> (VISA resource name out=w385:refnum<visa-resource-name>, error out=w384:errorcluster)  [unwired: 1 in, 1 out]
                  n172 = Wait (ms)(milliseconds to wait="读取间隔（毫秒）") -> ()  [unwired: 1 out]
                  n173 = Tick Count (ms)() -> (millisecond timer value=w392:u32)
                  n174 = call-by-ref "?"("nCount"=i16 1, "pValue"=w394, "nAxisNum"=3) -> ("pValue out"=w383:dbl)  [unwired: 7 in, 5 out]
                  n175 = Subtract(x=w392, y=w391) -> (x-y=w382:u32)
                }
                frame #1 {
                  n176 = Divide(x=w398, y=1000.0) -> (x/y=w397:dbl)
                  n177 = property class="Instr"(reference=w409, error in=w408) -> (reference out=w413:refnum<visa-resource-name>, error out=w423:errorcluster, "Serial Settings:Number of Bytes at Serial Port"=w414:u32)
                  n178 = Multiply(x=w397, y=0.078125) -> (x*y=→"位置(pluse)" →"位置" →"位移 2":dbl)
                  n179 = VISA Read(VISA resource name=w411, byte count=u32 128 ("字节总数"), error in (no error)=w410) -> (VISA resource name out=w404:refnum<visa-resource-name>, read buffer=w424:string, error out=w403:errorcluster)  [unwired: 1 out]
                  n180 = VISA Read(VISA resource name=w413, byte count=w414, error in (no error)=w423) -> (VISA resource name out=w405:refnum<visa-resource-name>, read buffer=w426:string, error out=w406:errorcluster)  [unwired: 1 out]
                  n181 = case shown="0, 默认" w402 {
                    tunnel: w424 -> [w429 w441]
                    frame 0, Default {
                      n182 = call <vilib>:"Delimited String to 1D String Array.vi"("delimiter"=",", "delimited string"=w429) -> ("string array"=w436:string[])  [unwired: 9 in]
                      n183 = Index Array(array=w436, index=0) -> (element=w431:string)
                      n184 = Index Array(array=w436, index=1) -> (element=w433:string)
                      n185 = Scan From String(input string=w431) -> (error out=w427:errorcluster, output 1=→"电感(H)" →"电阻表 3" →"电感":dbl)  [unwired: 4 in, 2 out]
                      n186 = Scan From String(input string=w433, error in=w427) -> (error out=→"错误输出":errorcluster, output 1=→"电阻(Ω)" →"电阻" →"电阻表 2":dbl)  [unwired: 3 in, 2 out]
                    }
                    frame 1 {
                      n187 = call <vilib>:"Delimited String to 1D String Array.vi"("delimiter"=",", "delimited string"=w441) -> ("string array"=w447:string[])  [unwired: 9 in]
                      n188 = Index Array(array=w447, index=0) -> (element=w440:string)
                      n189 = Index Array(array=w447, index=1) -> (element=w444:string)
                      n190 = Scan From String(input string=w440) -> (error out=w438:errorcluster, output 1=→"电容(F)" →"电容表" →"电容":dbl)  [unwired: 4 in, 2 out]
                      n191 = Scan From String(input string=w444, error in=w438) -> (error out=→"错误输出 2":errorcluster, output 1=→"损耗因子(F)" →"损耗因子" →"损耗因子表":dbl)  [unwired: 3 in, 2 out]
                    }
                  }
                  n192 = String Subset(string=w426, offset (0)=5 ("偏移量(0)"), length (rest)=2 ("长度（剩余）")) -> (substring=w417:string)
                  n193 = To Word Integer(number=0) -> (16bit integer=w419:i16)
                  n194 = Type Cast(type=w419, x=w417) -> (*(type *) &x=w420:i16)
                  n195 = Divide(x=w420, y=i16 10) -> (x/y=→"压力(g)" →"压力" →"压力表":dbl)
                  n196 = Wait (ms)(milliseconds to wait=u32 2 ("等待时间（毫秒）")) -> ()  [unwired: 1 out]
                  "时间" <- w407
                  "毫秒计时" <- w407
                }
              }
            }
            n197 = case shown="真" w354 {
              frame False {
              }
              frame True {
                n198 = invoke on="开始采集" class="Bool (严格)" method="Reinit To Default"() -> ()  [unwired: 3 in, 3 out]
                n199 = invoke on="采集状态" class="Bool (严格)" method="Reinit To Default"() -> ()  [unwired: 3 in, 3 out]
                n200 = invoke on="毫秒计时" class="DigNum (严格)" method="Reinit To Default"() -> ()  [unwired: 3 in, 3 out]
              }
            }
          }
        }
        "采集状态" <- "开始采集"
      }
      n201 = VISA Close(VISA resource name=w298, error in (no error)=w297) -> ()  [unwired: 1 out]
      n202 = VISA Close(VISA resource name=w296, error in (no error)=w295) -> ()  [unwired: 1 out]
    }
  }
  n203 = flat-sequence {
    frame #0 {
      n204 = Wait (ms)(milliseconds to wait=u32 500 ("等待时间（毫秒）")) -> ()  [unwired: 1 out]
    }
    frame #1 {
      n205 = while {
        stop <- FALSE stop-if-true
        w450 = 1000
        w460 = 0.078125 ("y")
        n206 = local read "目标位置(mm or °)"() -> (w467:dbl)
        n207 = local read "目标位置(mm or °)"() -> (w476:dbl)
        n208 = local read "目标位置(mm or °)"() -> (w473:dbl)
        n209 = local read "目标位置(mm or °)"() -> (w470:dbl)
        n210 = call-by-ref "?"("nCount"=i16 1, "pValue"=w476, "nAxisNum"=i16 1) -> ("pValue out"=w458:dbl)  [unwired: 7 in, 5 out]
        n211 = call-by-ref "?"("nCount"=i16 1, "pValue"=w473, "nAxisNum"=i16 2) -> ("pValue out"=w456:dbl)  [unwired: 7 in, 5 out]
        n212 = call-by-ref "?"("nCount"=i16 1, "pValue"=w470, "nAxisNum"=i16 3) -> ("pValue out"=w454:dbl)  [unwired: 7 in, 5 out]
        n213 = call-by-ref "?"("nCount"=i16 1, "pValue"=w467, "nAxisNum"=i16 4) -> ("pValue out"=w451:dbl)  [unwired: 7 in, 5 out]
        n214 = Divide(x=w451, y=w450) -> (x/y=w452:dbl)
        n215 = Divide(x=w456, y=w450) -> (x/y=w455:dbl)
        n216 = Divide(x=w458, y=w450) -> (x/y=w457:dbl)
        n217 = Divide(x=w454, y=w450) -> (x/y=w453:dbl)
        n218 = Multiply(x=w457, y=w460) -> (x*y=→"X":dbl)
        n219 = Multiply(x=w452, y=0.078125) -> (x*y=→"U":dbl)
        n220 = Multiply(x=w455, y=w460) -> (x*y=→"Y":dbl)
        n221 = Multiply(x=w453, y=w460) -> (x*y=→"Z":dbl)
      }
    }
  }
  "info" <- "" ("info")
